vi "SENS_SEGM_SWE_POIN.vi"(0 "VISA IN":refnum<visa-resource-name>, 1 "Segment":i32, 2 "Num Points":i32, 5 "error in":errorcluster, 7 "Channel":i32) -> (14 "VISA Out":refnum<visa-resource-name>, 19 "error out":errorcluster)   [LabVIEW 2018, in "PNA-X.lvlib"]
doc: "SENSe<cnum>:SEGMent<snum>:SWEep:POINts <num> \n1812\n\n(Read-Write) Sets the number of data points for the specified sweep segment. \nParameters \n<cnum> Any existing channel number. If unspecified, value is set to 1 \n<snum> Any existing segment number. If unspecified, value is set to 1 \n<num> Number of points in the segment. The total number of points in all segments \ncannot exceed 16001. A segment can have as few as 1 point. \nNote: This command will accept MIN or MAX instead of a numeric parameter. \nSee SCPI Syntax for more information. \nExamples SENS:SEGM:SWE:POIN 51 \nsense2:segment2:sweep:points maximum \nQuery Syntax SENSe<cnum>:SEGMent<snum>:SWEep:POINts? \nReturn Type Numeric \nDefault 21"
uses:
  PNA-X.lvlib
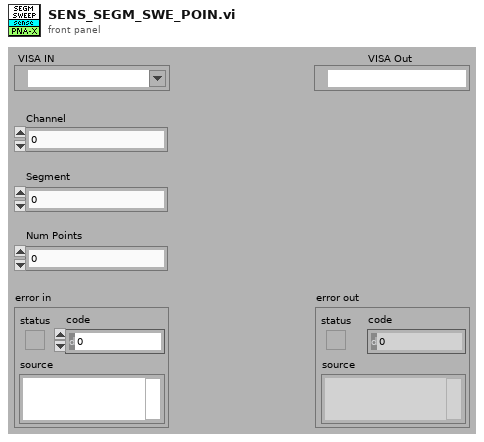
[diagram p1: front panel]
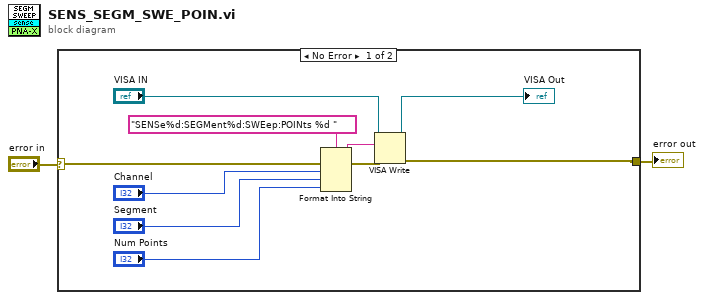
[diagram p0: block diagram]
diagram:
  n1 = case shown="No Error" "error in" {
    selector: "error in" -> [w12 w13]
    tunnel: [w7 w13] -> w1
    frame No Error {
      n2 = Format Into String(format string="SENSe%d:SEGMent%d:SWEep:POINts %d " ("Cmdline"), error in=w12, "Channel", "Segment", "Num Points") -> (resulting string=w10:string, error out=w11:errorcluster)  [unwired: 1 in]
      n3 = VISA Write(VISA resource name="VISA IN", write buffer=w10, error in (no error)=w11) -> (VISA resource name out=→"VISA Out":refnum<visa-resource-name>, error out=w7:errorcluster)  [unwired: 1 out]
    }
    frame Error {
    }
  }
  "error out" <- w1
